vi "4SpotScanTest.vi"() -> ()   [LabVIEW 2012]
uses:
  <userlib>/atmcd32d.llb/ReadMode_mode typedef.ctl
  <userlib>/atmcd32d.llb/AcquisitionMode_mode typedef.ctl
  <userlib>/atmcd32d.llb/TriggerMode_mode typedef.ctl
  <userlib>/atmcd32d.llb/Spool_method typedef.ctl
panel:
  out "Acquire":bool
  out "PannelClicked":bool
  out "CurrentPannel":u16
  out "Pos_4":cluster{"X":dbl, "Y":dbl}
  out "Pos_3":cluster{"X":dbl, "Y":dbl}
  out "Pos_2":cluster{"X":dbl, "Y":dbl}
  out "Pos_1":cluster{"X":dbl, "Y":dbl}
  out "MousePos":cluster{"X":dbl, "Y":dbl}
  out "Amp":T1(graph)
  out "SubImage_DownRight":u16[][](graph)
  out "SubImage_DownLeft":u16[][](graph)
  out "SubImage_UpRight":u16[][](graph)
  out "SubImage_UpLeft":u16[][](graph)
  in  "Stop":bool
  out "CurrentPosition":dbl
  out "acq count":dbl
  in  "channel":string
  in  "start":dbl
  in  "cycle":dbl
  in  "Path":path=path "e:/"
  in  "File Name":string="scan"
  in  "START SCAN":bool
  in  "Frame":dbl
  in  "Delay":dbl
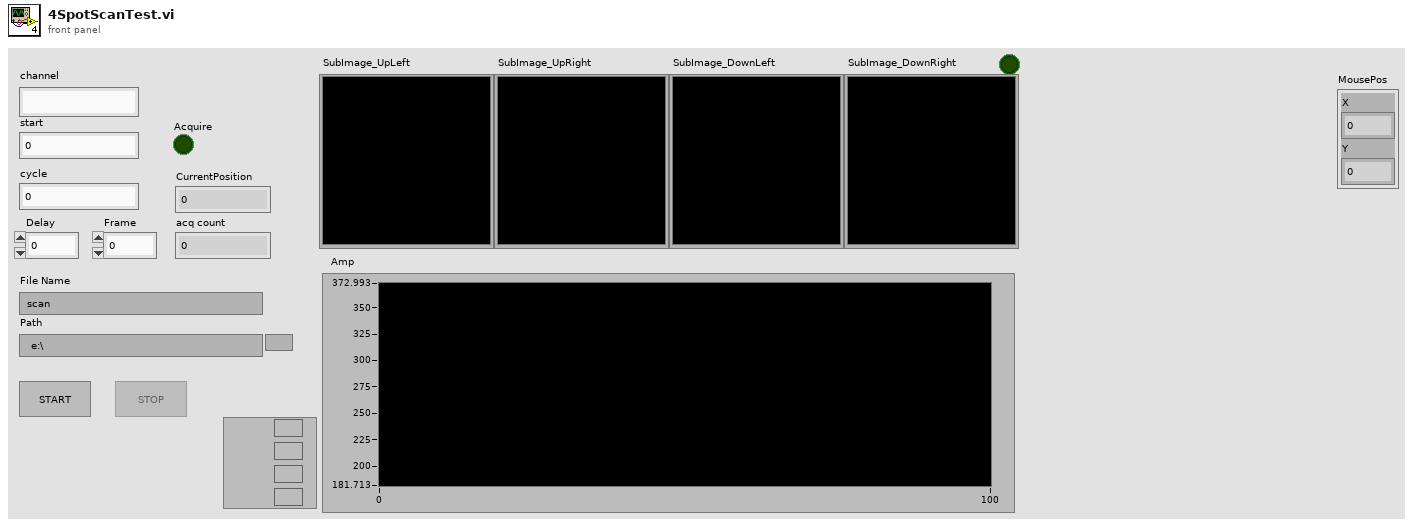
[diagram p1: front panel]
types:
  T1 = cluster{"UpLeft":dbl, "UpRight":dbl, "DownLeft":dbl, "DownRight":dbl}
  T2 = cluster{"image":i16[][], "x_start":u32, "x_end":u32, "y_start":u32, "y_end":u32, "ImageCnt":u32, "subImage":u16[][]}
  T3 = cluster{"Amp":dbl, "PosX":dbl, "PosY":dbl, "StdX":dbl, "StdY":dbl, "Bkg":dbl, "Steps":i32, "time":dbl}
  T4 = enum8{"Enabled", "Disabled", "Disabled and Grayed Out"}
  T5 = typedef "ReadMode_mode typedef.ctl" = enum16{"Full Vertical Binning", "Multi-Track", "Random-Track", "Single-Track", "Image"}
  T6 = typedef "AcquisitionMode_mode typedef.ctl" = enum16{"Reserved (0)", "Single Scan", "Accumulate", "Kinetics", "Fast Kinetics", "Run Till Abort", "Reserved (6)", "Reserved (7)", "Reserved (8)", "Time Delayed Integration"}
  T7 = typedef "TriggerMode_mode typedef.ctl" = enum16{"Internal", "External", "N/A (2)", "N/A (3)", "N/A (4)", "N/A (5)", "External Start", "External Exposure (Bulb)", "N/A (8)", "External FVB EM", "Software", "N/A (11)", "External Charge Shifting"}
  T8 = typedef "Spool_method typedef.ctl" = enum16{"32-bit", "Depends", "16-bit", "Multiple Directory", "Spool to RAM disk", "16-bit FITS", "SIF", "16-buit TIFF", "Multiple Directory Compressed"}
  T9 = cluster{"UpLeft":dbl, "UpRight":dbl, "DownLeft":dbl, "DownRight":dbl}[]
  T10 = cluster{"DeviceID":string, "Channel":string, "param1":dbl, "Operation":string}
  T11 = cluster{"Position":cluster{"X":dbl, "Y":dbl}, "DoubleClick":bool}
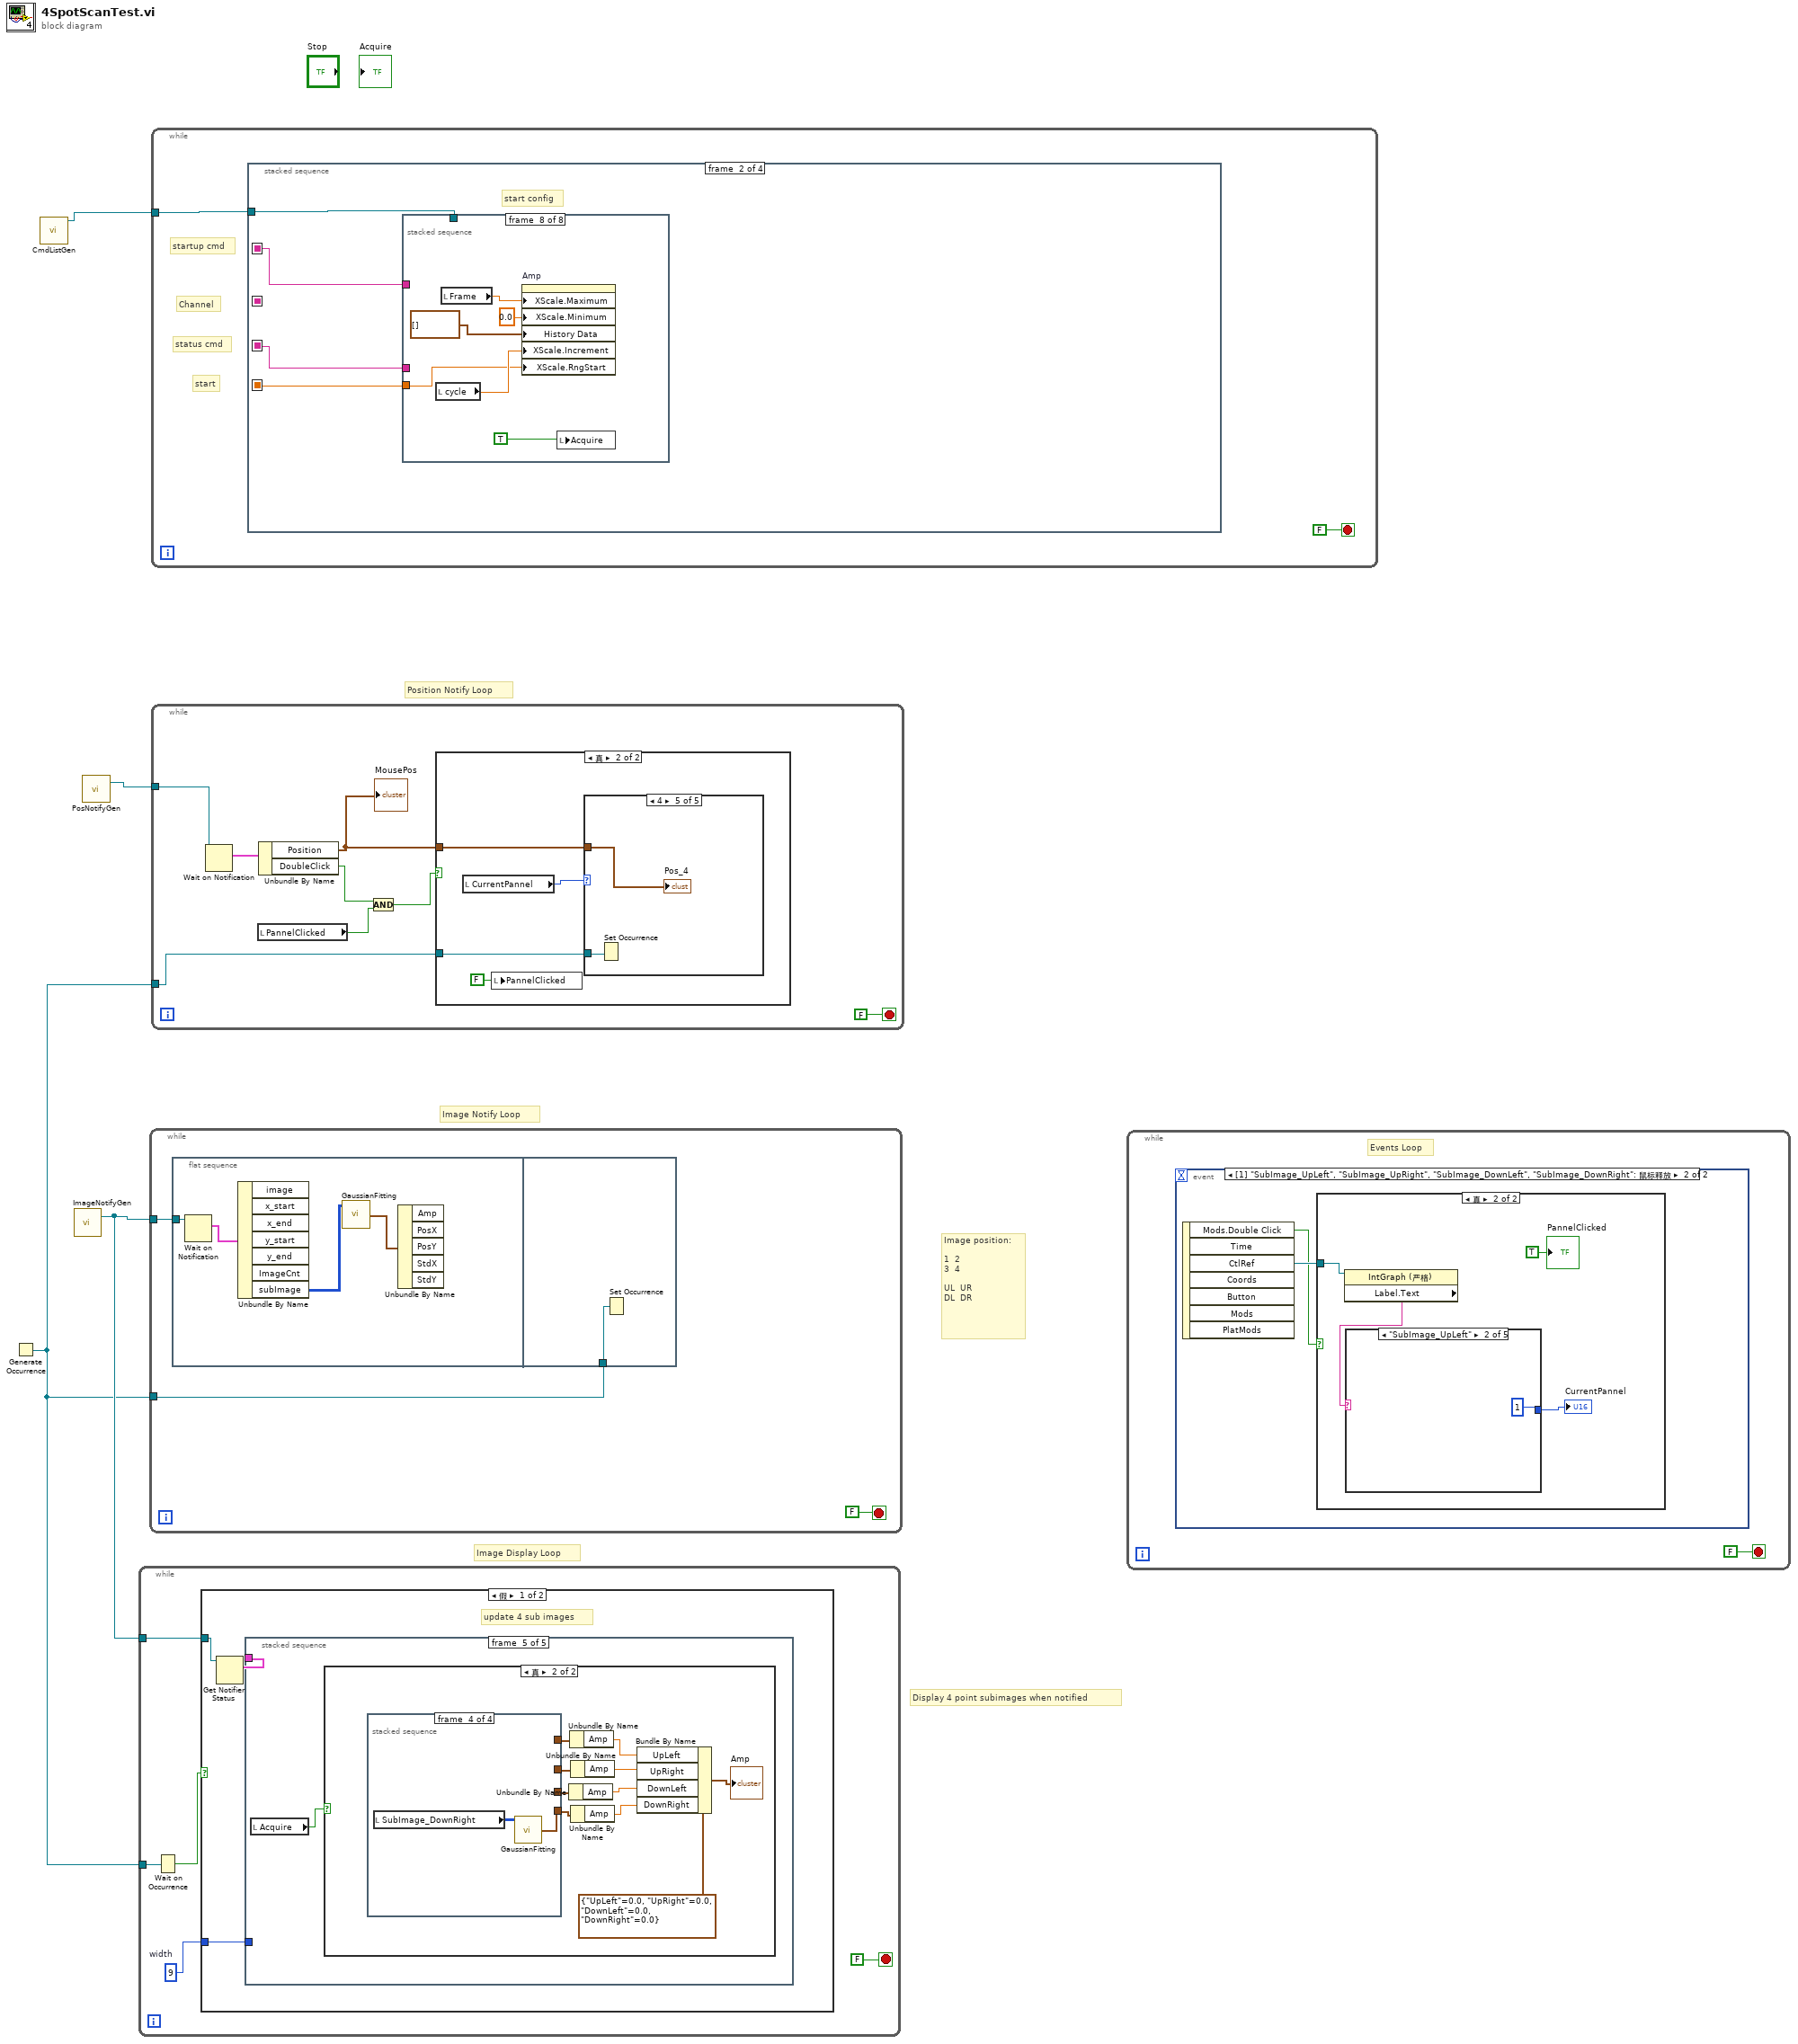
[diagram p0: block diagram]
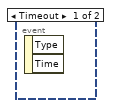
[diagram p2: hidden frame]
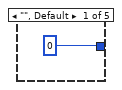
[diagram p4: hidden frame]
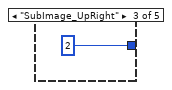
[diagram p5: hidden frame]
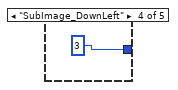
[diagram p6: hidden frame]
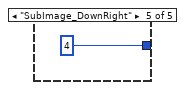
[diagram p7: hidden frame]
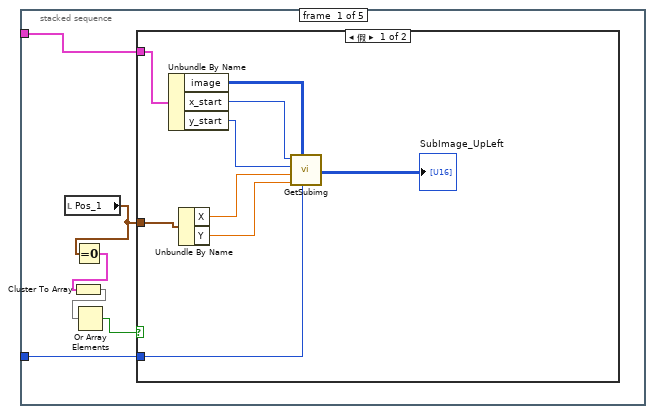
[diagram p8: hidden frame]
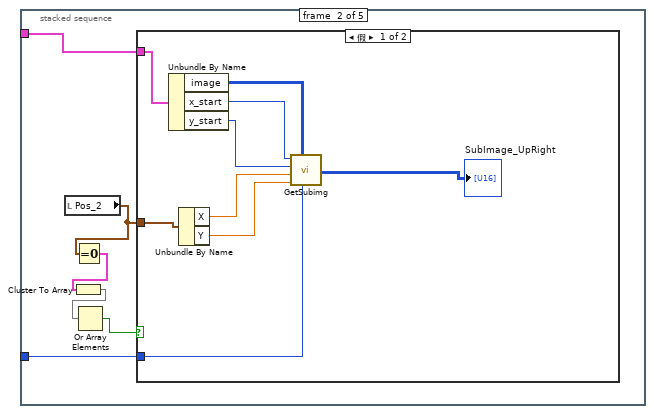
[diagram p10: hidden frame]
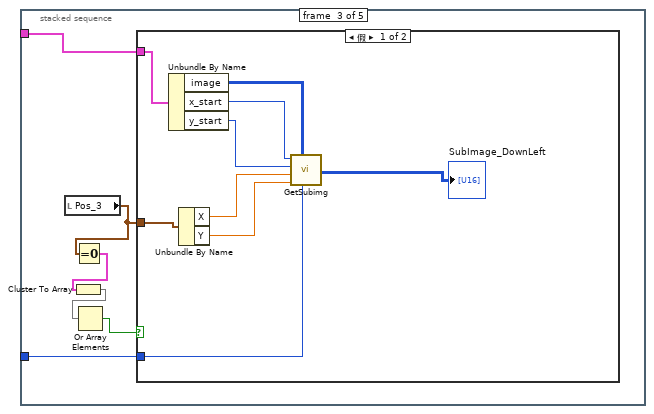
[diagram p12: hidden frame]
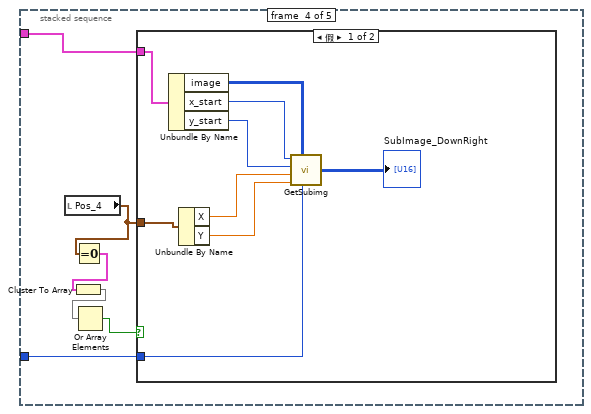
[diagram p14: hidden frame]
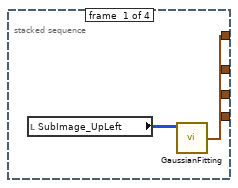
[diagram p17: hidden frame]
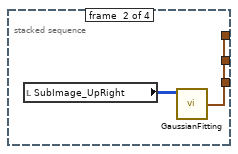
[diagram p18: hidden frame]
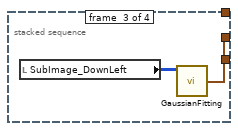
[diagram p19: hidden frame]
diagram:
  # "Display 4 point subimages when notified"
  # "Image position:\n\n1  2\n3  4\n\nUL  UR\nDL  DR"
  # "Image Display Loop"
  # "Image Notify Loop"
  # "Position Notify Loop"
  n1 = Generate Occurrence() -> (w1:refnum<k4>)
  n2 = call "CmdListGen.vi"() -> ("MsgList"=w4:refnum<queue>)  [unwired: 1 in, 3 out]
  n3 = call "ImageNotifyGen.vi"() -> ("ImageNotifyRef"=w2:refnum<notifier>)  [unwired: 2 in, 1 out]
  n4 = call "PosNotifyGen.vi"() -> ("NotifyRef"=w3:refnum<notifier>)  [unwired: 2 in, 1 out]
  n5 = while {
    tunnel: w2 -> [w5]
    tunnel: w1 -> [w8]
    stop <- FALSE stop-if-true
    w6 = 9  # width
    n6 = Wait on Occurrence(2:w8) -> (0:w7:bool)  [unwired: 2 in]
    n7 = case shown="假" w7 {
      tunnel: w6 -> [w12 _]
      tunnel: w5 -> [w10 _]
      frame False {
        # "update 4 sub images"
        n8 = Get Notifier Status(notifier=w10) -> (current notification=w11:T2)  [unwired: 1 in, 4 out]
        n9 = stacked-sequence {
          tunnel: w11 -> [w14 w29 w44 w59 _]
          tunnel: w12 -> [w13 w28 w43 w58 _]
          frame #0 {
            n10 = local read "Pos_1"() -> (w18:cluster{"X":dbl, "Y":dbl})
            n11 = Equal To 0?(x=w18) -> (x = 0?=w17:cluster{"X":bool, "Y":bool})
            n12 = Cluster To Array(cluster=w17) -> (array=w16:bool[])
            n13 = Or Array Elements(Boolean array=w16) -> (logical OR=w15:bool)
            n14 = case shown="假" w15 {
              tunnel: w18 -> [w27 _]
              tunnel: w14 -> [w26 _]
              tunnel: w13 -> [w20 _]
              frame False {
                n15 = Unbundle By Name(w26) -> ("image"=w25:i16[][], "x_start"=w24:u32, "y_start"=w23:u32)
                n16 = Unbundle By Name(w27) -> ("X"=w22:dbl, "Y"=w21:dbl)
                n17 = call "GetSubimg.vi"("width"=w20, "Img in"=w25, "y"=w21, "x"=w22, "y_start"=w23, "x_start"=w24) -> ("SubImage"=→"SubImage_UpLeft":u16[][])
              }
              frame True {
              }
            }
          }
          frame #1 {
            n18 = local read "Pos_2"() -> (w33:cluster{"X":dbl, "Y":dbl})
            n19 = Equal To 0?(x=w33) -> (x = 0?=w32:cluster{"X":bool, "Y":bool})
            n20 = Cluster To Array(cluster=w32) -> (array=w31:bool[])
            n21 = Or Array Elements(Boolean array=w31) -> (logical OR=w30:bool)
            n22 = case shown="假" w30 {
              tunnel: w33 -> [w42 _]
              tunnel: w29 -> [w41 _]
              tunnel: w28 -> [w35 _]
              frame False {
                n23 = Unbundle By Name(w41) -> ("image"=w40:i16[][], "x_start"=w39:u32, "y_start"=w38:u32)
                n24 = Unbundle By Name(w42) -> ("X"=w37:dbl, "Y"=w36:dbl)
                n25 = call "GetSubimg.vi"("width"=w35, "Img in"=w40, "y"=w36, "x"=w37, "y_start"=w38, "x_start"=w39) -> ("SubImage"=→"SubImage_UpRight":u16[][])
              }
              frame True {
              }
            }
          }
          frame #2 {
            n26 = local read "Pos_3"() -> (w48:cluster{"X":dbl, "Y":dbl})
            n27 = Equal To 0?(x=w48) -> (x = 0?=w47:cluster{"X":bool, "Y":bool})
            n28 = Cluster To Array(cluster=w47) -> (array=w46:bool[])
            n29 = Or Array Elements(Boolean array=w46) -> (logical OR=w45:bool)
            n30 = case shown="假" w45 {
              tunnel: w48 -> [w57 _]
              tunnel: w44 -> [w56 _]
              tunnel: w43 -> [w50 _]
              frame False {
                n31 = Unbundle By Name(w56) -> ("image"=w55:i16[][], "x_start"=w54:u32, "y_start"=w53:u32)
                n32 = Unbundle By Name(w57) -> ("X"=w52:dbl, "Y"=w51:dbl)
                n33 = call "GetSubimg.vi"("width"=w50, "Img in"=w55, "y"=w51, "x"=w52, "y_start"=w53, "x_start"=w54) -> ("SubImage"=→"SubImage_DownLeft":u16[][])
              }
              frame True {
              }
            }
          }
          frame #3 {
            n34 = local read "Pos_4"() -> (w63:cluster{"X":dbl, "Y":dbl})
            n35 = Equal To 0?(x=w63) -> (x = 0?=w62:cluster{"X":bool, "Y":bool})
            n36 = Cluster To Array(cluster=w62) -> (array=w61:bool[])
            n37 = Or Array Elements(Boolean array=w61) -> (logical OR=w60:bool)
            n38 = case shown="假" w60 {
              tunnel: w63 -> [w72 _]
              tunnel: w59 -> [w71 _]
              tunnel: w58 -> [w65 _]
              frame False {
                n39 = Unbundle By Name(w71) -> ("image"=w70:i16[][], "x_start"=w69:u32, "y_start"=w68:u32)
                n40 = Unbundle By Name(w72) -> ("X"=w67:dbl, "Y"=w66:dbl)
                n41 = call "GetSubimg.vi"("width"=w65, "Img in"=w70, "y"=w66, "x"=w67, "y_start"=w68, "x_start"=w69) -> ("SubImage"=→"SubImage_DownRight":u16[][])
              }
              frame True {
              }
            }
          }
          frame #4 {
            n42 = local read "Acquire"() -> (w73:bool)
            n43 = case shown="真" w73 {
              frame False {
              }
              frame True {
                n44 = stacked-sequence {
                  tunnel: [w84 _ _ _] -> w83
                  tunnel: [_ w86 _ _] -> w82
                  tunnel: [_ _ w88 _] -> w81
                  tunnel: [_ _ _ w90] -> w80
                  frame #0 {
                    n45 = local read "SubImage_UpLeft"() -> (w85:u16[][])
                    n46 = call "GaussianFitting.vi"("数组"=w85) -> ("Result"=w84:T3)  [unwired: 2 in]
                  }
                  frame #1 {
                    n47 = local read "SubImage_UpRight"() -> (w87:u16[][])
                    n48 = call "GaussianFitting.vi"("数组"=w87) -> ("Result"=w86:T3)  [unwired: 2 in]
                  }
                  frame #2 {
                    n49 = local read "SubImage_DownLeft"() -> (w89:u16[][])
                    n50 = call "GaussianFitting.vi"("数组"=w89) -> ("Result"=w88:T3)  [unwired: 2 in]
                  }
                  frame #3 {
                    n51 = local read "SubImage_DownRight"() -> (w91:u16[][])
                    n52 = call "GaussianFitting.vi"("数组"=w91) -> ("Result"=w90:T3)  [unwired: 2 in]
                  }
                }
                n53 = Unbundle By Name(w81) -> ("Amp"=w76:dbl)
                n54 = Unbundle By Name(w83) -> ("Amp"=w78:dbl)
                n55 = Unbundle By Name(w82) -> ("Amp"=w77:dbl)
                n56 = Unbundle By Name(w80) -> ("Amp"=w75:dbl)
                n57 = Bundle By Name(cluster=T1 {"UpLeft"=0.0, "UpRight"=0.0, "DownLeft"=0.0, "DownRight"=0.0} ("输入簇"), "UpLeft"=w78, "UpRight"=w77, "DownLeft"=w76, "DownRight"=w75) -> (→"Amp":T1)
              }
            }
          }
        }
      }
      frame True {
      }
    }
  }
  n58 = while {
    tunnel: w2 -> [w94]
    tunnel: w1 -> [w92]
    stop <- FALSE ("停止") stop-if-true
    n59 = flat-sequence {
      tunnel: w94 -> [w98]
      tunnel: w92 -> [w99]
      frame #0 {
        n60 = Wait on Notification(notifier=w98) -> (notification=w97:T2)  [unwired: 3 in, 3 out]
        n61 = Unbundle By Name(w97) -> ("subImage"=w95:u16[][])  [unwired: 6 out]
        n62 = call "GaussianFitting.vi"("数组"=w95) -> ("Result"=w96:T3)  [unwired: 2 in]
        n63 = Unbundle By Name(w96) -> ()  [unwired: 5 out]
      }
      frame #1 {
        n64 = Set Occurrence(w99) -> ()
      }
    }
  }
  n65 = while {
    tunnel: w4 -> [w100]
    stop <- FALSE stop-if-true
    # "status cmd"
    # "Channel"
    # "startup cmd"
    # "start"
    n66 = stacked-sequence {
      seq-local: [w105 _ _ _] -> [_ w120 _ _]
      seq-local: [w104 _ _ _] -> [_ _ w148 _]
      seq-local: [w103 _ _ _] -> [_ w119 w147 _]
      seq-local: [w102 _ _ _] -> [_ w118 w146 _]
      tunnel: w100 -> [_ w121 w149 _]
      frame #0 {
        # "wait for start"
        n67 = flat-sequence {
          tunnel: [w115] -> w105
          tunnel: ["channel"] -> w104
          tunnel: [w113] -> w103
          tunnel: ["start"] -> w102
          frame #0 {
            n68 = property on="START SCAN" class="Bool"("DisabledEnum"=T4."Enabled" ("禁用")) -> ()  [unwired: 2 in, 2 out]
            n69 = property on="Stop" class="Bool (严格)"("DisabledEnum"=T4."Disabled and Grayed Out" ("禁用")) -> ()  [unwired: 2 in, 2 out]
          }
          frame #1 {
            n70 = while {
              stop <- "START SCAN" stop-if-true
              n71 = Wait Until Next ms Multiple(millisecond multiple=u32 50 ("毫秒倍数")) -> ()  [unwired: 1 out]
            }
          }
          frame #2 {
            n72 = property on="START SCAN" class="Bool"("DisabledEnum"=T4."Disabled and Grayed Out" ("禁用")) -> ()  [unwired: 2 in, 2 out]
            n73 = property on="Stop" class="Bool (严格)"("DisabledEnum"=T4."Enabled" ("禁用")) -> ()  [unwired: 2 in, 2 out]
          }
          frame #3 {
            # "status cmd"
            # "startup cmd"
            n74 = Concatenate Strings("channel", ",GETS,0" ("格式字符串")) -> (w113:string)
            n75 = Format Into String(format string="%s,MOVP,%f" ("格式字符串"), "channel", "start") -> (resulting string=w115:string)  [unwired: 2 in, 1 out]
          }
        }
      }
      frame #1 {
        # "start config"
        n76 = stacked-sequence {
          tunnel: w121 -> [w123 w125 _ _ _ _ _ _]
          tunnel: w120 -> [w122 _ _ _ _ _ _ _]
          tunnel: w119 -> [_ w124 _ _ _ _ _ _]
          tunnel: w118 -> [_ _ _ _ _ _ _ w140]
          frame #0 {
            n77 = call "PassCmd.vi"("cmd in"=w122, "list ref"=w123) -> ()  [unwired: 1 in, 2 out]
          }
          frame #1 {
            n78 = while {
              tunnel: w125 -> [w131]
              tunnel: w124 -> [w126]
              stop <- w127 stop-if-true
              n79 = call "PassCmd.vi"("cmd in"=w126, "list ref"=w131) -> ("str out"=w130:string)  [unwired: 1 in, 1 out]
              n80 = call "str2code.vi"("input"=w130) -> ("Output"=w129:T10)  [unwired: 1 in, 1 out]
              n81 = Unbundle By Name(w129) -> ("param1"=w128:dbl)
              n82 = Equal To 0?(x=w128) -> (x = 0?=w127:bool)
            }
          }
          frame #2 {
            n83 = call <userlib>:"SetReadMode.vi"("mode"=ReadMode_mode_typedef."Image") -> ()  [unwired: 1 in, 2 out]
          }
          frame #3 {
            n84 = call <userlib>:"SetAcquisitionMode.vi"("mode"=AcquisitionMode_mode_typedef."Run Till Abort") -> ()  [unwired: 1 in, 2 out]
          }
          frame #4 {
            n85 = call <userlib>:"SetTriggerMode.vi"("mode"=TriggerMode_mode_typedef."Software") -> ()  [unwired: 1 in, 2 out]
          }
          frame #5 {
            n86 = call "path.vi"("file"="File Name", "path_in"="Path") -> ("path_out"=w135:string)
            n87 = call <userlib>:"SetSpool.vi"("active"=TRUE, "method"=Spool_method_typedef."16-buit TIFF", "name"=w135) -> ()  [unwired: 11 in, 2 out]
          }
          frame #6 {
            n88 = call <userlib>:"StartAcquisition.vi"() -> ()  [unwired: 2 in, 2 out]
          }
          frame #7 {
            n89 = local read "cycle"() -> (w141:dbl)
            n90 = local read "Frame"() -> (w144:dbl)
            n91 = property on="Amp" class="WFChart (严格)"("XScale.Maximum"=w144, "XScale.Minimum"=0.0 ("X标尺.范围:最小值"), "History Data"=T9 [] ("历史数据"), "XScale.Increment"=w141, "XScale.RngStart"=w140) -> ()  [unwired: 2 in, 2 out]
            n92 = local write "Acquire"(TRUE) -> ()
          }
        }
      }
      frame #2 {
        # "Acquisition"
        n93 = for {
          N: "Frame" -> [_]
          tunnel: w149 -> [w162]
          shift-right: [w159] -> _
          shift-left: _ -> [w160]
          shift-right: [w152] -> _
          shift-left: w146 -> [w156]
          tunnel: w147 -> [w158]
          tunnel: w148 -> [w157]
          i -> [w153]
          stop <- w151 stop-if-true
          n94 = Increment(x=w153) -> (x+1=→"acq count":i32)
          n95 = Add(x=w156, y="cycle") -> (x+y=w152:dbl)
          n96 = stacked-sequence {
            tunnel: w162 -> [w164 w174 _ _ w198]
            tunnel: w160 -> [_ _ _ w184 _]
            tunnel: [_ _ _ w185 _] -> w159
            tunnel: w158 -> [w163 _ _ _ _]
            tunnel: w152 -> [_ _ _ _ w196]
            tunnel: w157 -> [_ w175 _ _ w197]
            frame #0 {
              n97 = while {
                tunnel: w164 -> [w172]
                tunnel: w163 -> [w168]
                stop <- w165 stop-if-true
                n98 = call "PassCmd.vi"("cmd in"=w168, "list ref"=w172) -> ("str out"=w171:string)  [unwired: 1 in, 1 out]
                n99 = local read "Stop"() -> (w166:bool)
                n100 = call "str2code.vi"("input"=w171) -> ("Output"=w170:T10)  [unwired: 1 in, 1 out]
                n101 = Unbundle By Name(w170) -> ("param1"=w169:dbl)
                n102 = Equal To 0?(x=w169) -> (x = 0?=w167:bool)
                n103 = Or(x=w167, y=w166) -> (x .or. y?=w165:bool)
              }
            }
            frame #1 {
              # "display position"
              n104 = local read "Stop"() -> (w173:bool)
              n105 = case shown="假" w173 {
                tunnel: w175 -> [_ w180]
                tunnel: w174 -> [_ w177]
                frame True {
                }
                frame False {
                  n106 = Concatenate Strings(w180, ",GETP,0" ("字符串")) -> (w178:string)
                  n107 = call "PassCmd.vi"("cmd in"=w178, "list ref"=w177) -> ("str out"=w182:string)  [unwired: 1 in, 1 out]
                  n108 = call "str2code.vi"("input"=w182) -> ("Output"=w181:T10)  [unwired: 1 in, 1 out]
                  n109 = Unbundle By Name(w181) -> ("param1"=→"CurrentPosition":dbl)
                }
              }
            }
            frame #2 {
              n110 = local read "Stop"() -> (w183:bool)
              n111 = case shown="假" w183 {
                frame True {
                }
                frame False {
                  n112 = call <userlib>:"SendSoftwareTrigger.vi"() -> ()  [unwired: 1 in, 2 out]
                }
              }
            }
            frame #3 {
              n113 = while {
                tunnel: w184 -> [w192]
                tunnel: [w189] -> w185
                stop <- w186 stop-if-true
                n114 = call <userlib>:"GetNumberNewImages.vi"() -> ("error out"=w191:errorcluster, "last"=w190:i32)  [unwired: 4 in, 2 out]
                n115 = local read "Stop"() -> (w187:bool)
                n116 = case shown="无错误" w191 {
                  tunnel: w190 -> [w193 _]
                  tunnel: [w193 0] -> w189
                  frame No Error {
                  }
                  frame Error {
                  }
                }
                n117 = Not Equal?(x=w189, y=w192) -> (x != y?=w188:bool)
                n118 = Or(x=w188, y=w187) -> (x .or. y?=w186:bool)
              }
            }
            frame #4 {
              n119 = local read "Stop"() -> (w195:bool)
              n120 = case shown="假" w195 {
                tunnel: w198 -> [_ w203]
                tunnel: w197 -> [_ w201]
                tunnel: w196 -> [_ w200]
                frame True {
                }
                frame False {
                  n121 = Format Into String(format string="%s,MOVP,%f" ("格式字符串"), w201, w200) -> (resulting string=w199:string)  [unwired: 2 in, 1 out]
                  n122 = call "PassCmd.vi"("cmd in"=w199, "list ref"=w203) -> ()  [unwired: 1 in, 2 out]
                }
              }
            }
          }
          n123 = Wait (ms)(milliseconds to wait="Delay") -> ()  [unwired: 1 out]
          n124 = local read "Stop"() -> (w151:bool)
        }
      }
      frame #3 {
        w204 = FALSE ("Stop")
        # "Stop Acquisition"
        n125 = local write "Stop"(w204) -> ()
        n126 = call <userlib>:"AbortAcquisition.vi"() -> ()  [unwired: 2 in, 2 out]
        n127 = local write "Acquire"(w204) -> ()
      }
    }
  }
  n128 = while {
    tunnel: w3 -> [w212]
    tunnel: w1 -> [w205]
    stop <- FALSE stop-if-true
    n129 = Wait on Notification(notifier=w212) -> (notification=w210:T11)  [unwired: 3 in, 3 out]
    n130 = local read "PannelClicked"() -> (w208:bool)
    n131 = Unbundle By Name(w210) -> ("Position"=w206:cluster{"X":dbl, "Y":dbl}, "DoubleClick"=w209:bool)
    "MousePos" <- w206
    n132 = And(x=w209, y=w208) -> (x .and. y?=w207:bool)
    n133 = case shown="真" w207 {
      tunnel: w206 -> [_ w215]
      tunnel: w205 -> [_ w214]
      frame False {
      }
      frame True {
        n134 = local read "CurrentPannel"() -> (w216:u16)
        n135 = local write "PannelClicked"(FALSE ("PannelClicked")) -> ()
        n136 = case shown="4" w216 {
          tunnel: w215 -> [_ w218 w220 w222 w224]
          tunnel: w214 -> [_ w217 w219 w221 w223]
          frame 0, Default {
          }
          frame 1 {
            n137 = Set Occurrence(w217) -> ()
            "Pos_1" <- w218
          }
          frame 2 {
            n138 = Set Occurrence(w219) -> ()
            "Pos_2" <- w220
          }
          frame 3 {
            n139 = Set Occurrence(w221) -> ()
            "Pos_3" <- w222
          }
          frame 4 {
            n140 = Set Occurrence(w223) -> ()
            "Pos_4" <- w224
          }
        }
      }
    }
  }
  n141 = while {
    stop <- FALSE stop-if-true
    # "Events Loop"
    n142 = event shown="[1] \"SubImage_UpLeft\", \"SubImage_UpRight\", \"SubImage_DownLeft\", \"SubImage_DownRight\": 鼠标释放" {
      selector: _ -> [_ _]
      dyn-events: _ -> [_ _]
      timeout: _ -> [_ _]
      event Timeout {
        n143 = event-data() -> ()  [unwired: 1 in, 2 out]
      }
      event "SubImage_UpLeft", "SubImage_UpRight", "SubImage_DownLeft", "SubImage_DownRight": Mouse Up {
        n144 = event-data() -> ("Mods.Double Click"=w226:bool, "CtlRef"=w227:refnum<vi>)  [unwired: 1 in, 5 out]
        n145 = case shown="真" w226 {
          tunnel: w227 -> [_ w228]
          frame False {
          }
          frame True {
            n146 = property class="IntGraph (严格)"(reference=w228) -> ("Label.Text"=w231:string)  [unwired: 1 in, 2 out]
            n147 = case shown="\"SubImage_UpLeft\"" w231 {
              tunnel: [0 1 2 3 4] -> w230
              frame "", Default {
              }
              frame "SubImage_UpLeft" {
              }
              frame "SubImage_UpRight" {
              }
              frame "SubImage_DownLeft" {
              }
              frame "SubImage_DownRight" {
              }
            }
            "CurrentPannel" <- w230
            "PannelClicked" <- TRUE ("PannelClicked")
          }
        }
      }
    }
  }
